vi "Write Configuration.vi"(8 "error in (no error)":errorcluster, 11 "connection string":string) -> (0 "error out":errorcluster)   [LabVIEW 2019, in "LV-Data.PGSQL.lvclass"]
uses:
  LV-Data.PGSQL.lvclass
  <vilib>/Utility/config.llb/Write Key (String).vi
  <vilib>/Utility/config.llb/NI_LVConfig.lvlib
panel:
  out "found?":bool
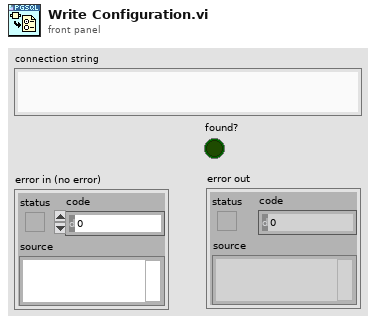
[diagram p1: front panel]
types:
  T1 = typedef "NI_LVConfig.lvlib/Config Data RefNum.ctl" = refnum<k1>
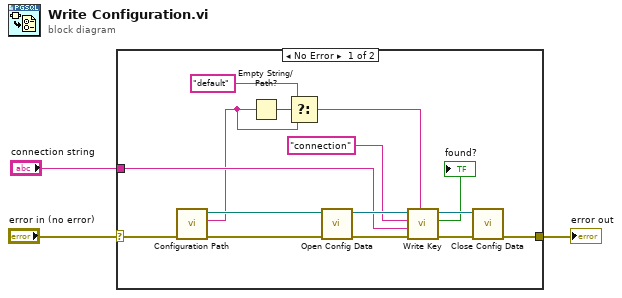
[diagram p0: block diagram]
diagram:
  n1 = case shown="No Error" "error in (no error)" {
    selector: "error in (no error)" -> [w18 w19]
    tunnel: [w17 w19] -> w3
    tunnel: "connection string" -> [w12 _]
    frame No Error {
      n2 = call "Configuration Path.vi"("error in (no error)"=w18) -> ("error out"=w16:errorcluster, "section"=w7:string, "path"=w15:path)  [unwired: 8 in]
      n3 = Empty String/Path?(string/path=w7) -> (empty?=w8:bool)
      n4 = Select(t="default" ("section"), s=w8, f=w7) -> (s? t:f=w5:string)
      n5 = call <vilib>:"Open Config Data.vi"("error in (no error)"=w16, "configuration file path"=w15) -> ("error out"=w14:errorcluster, "refnum"=w13:T1)  [unwired: 7 in, 1 out]
      n6 = call-poly <vilib>:"Write Key.vi"("section"=w5, "error in (no error)"=w14, "value"=w12, "key"="connection", "refnum"=w13) -> ("error out"=w10:errorcluster, "found?"=→"found?":bool, "refnum out"=w11:T1)  [unwired: 4 in]
      n7 = call <vilib>:"Close Config Data.vi"("error in (no error)"=w10, "refnum"=w11) -> ("error out"=w17:errorcluster)  [unwired: 8 in, 1 out]
    }
    frame Error {
    }
  }
  "error out" <- w3
